vi "VIRBdll.vi"(8 "error in (no error)":errorcluster, 10 "z":dbl[](array[numeric]), 11 "t":dbl) -> (0 "error out":errorcluster, 3 "b out":dbl)   [LabVIEW 2016]
doc: "subroutine VIRB (t,z, b)\n\ncompute second virial coefficient as a function of temperature and composition.\n\nINPUTS:\n t--temperature [K]\n z--composition [array of mol frac]\nOUTPUTS:\n b--second virial coefficient [L/mol]"
uses:
  REFPROP.DLL
panel:
  # "REFPROP-VIRBdll.vi"
  # "void  VIRBdll(double *t, double *z, double *b)"
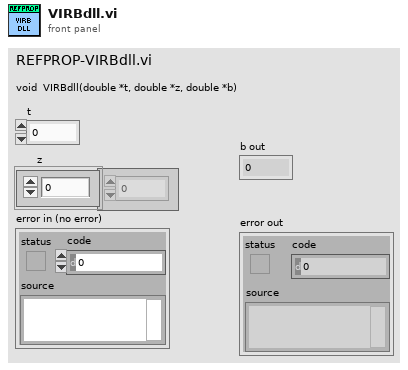
[diagram p1: front panel]
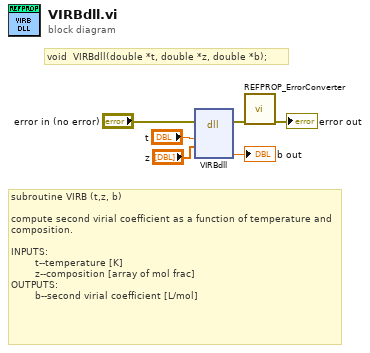
[diagram p0: block diagram]
diagram:
  # "void  VIRBdll(double *t, double *z, double *b);"
  # "subroutine VIRB (t,z, b)\n\ncompute second virial coefficient as a function of temperature and composition.\n\nINPUTS:\n        t--temperature [K]\n        z--composition [array of mol frac]\nOUTPUTS:\n        b--second virial coefficient [L/mol]"
  n1 = dll-call lib="S:/009 - Testing/02 - Performance Testing/REFPROP/REFPROP.*" fn="VIRBdll"(error in="error in (no error)", "t"="t", "z"="z") -> (error out=w3:errorcluster, "b"=→"b out":dbl)  [unwired: 6 in, 1 out]
  n2 = call "REFPROP_ErrorConverter.vi"("error in (no error)"=w3) -> ("error out"=→"error out":errorcluster)  [unwired: 10 in]
